vi "Configure.vi"(10 "CfgIn":T8={"Baud Rate"=enum."9600 bps", "Baud Rate Divider"=192, "Prescaler"=enum."1", "Data Bits"=enum."8", "Stop Bits"=enum."1", "Parity"=enum."None", "Flow Control"=enum."None", "Transceiver Mode"=enum."4 Wire"}, 11 "Serial FPGA in":refnum<class "Serial FPGA.lvclass">) -> (3 "Serial FPGA out":refnum<class "Serial FPGA.lvclass">)   [LabVIEW 2013, in "Serial FPGA.lvclass"]
uses:
  Serial FPGA.lvclass
  <vilib>/LabVIEW Targets/FPGA/cRIO/shared/nicrio_ModuleControls/nicrio_cRIO-9871_BaudRateEnum.ctl
  <vilib>/LabVIEW Targets/FPGA/cRIO/shared/nicrio_ModuleControls/nicrio_cRIO-9871_BaudRatePrescalerEnum.ctl
  <vilib>/LabVIEW Targets/FPGA/cRIO/shared/nicrio_ModuleControls/nicrio_cRIO-9871_DataBitsEnum.ctl
  <vilib>/LabVIEW Targets/FPGA/cRIO/shared/nicrio_ModuleControls/nicrio_cRIO-9871_StopBitsEnum.ctl
  <vilib>/LabVIEW Targets/FPGA/cRIO/shared/nicrio_ModuleControls/nicrio_cRIO-9871_ParityEnum.ctl
  <vilib>/LabVIEW Targets/FPGA/cRIO/shared/nicrio_ModuleControls/nicrio_cRIO-9871_FlowControlEnum.ctl
  <vilib>/LabVIEW Targets/FPGA/cRIO/shared/nicrio_ModuleControls/nicrio_cRIO-9871_XcvrModeEnum.ctl
  Serial FPGA.lvclass/Serial FPGA.ctl
  <vilib>/rvi/eio/common/nirviEmuTemplatePropertySet_noerrors.vi
  <vilib>/eio/EIOPropertyNode/EIOPropertyNode.xnode
  <vilib>/rvi/eio/common/nirviEmuTemplatePropertyGet_errors.vi
  <vilib>/rvi/eio/common/nirviEmuTemplatePropertyGet_noerrors.vi
  <vilib>/rvi/eio/common/nirviEmuTemplatePropertySet_errors.vi
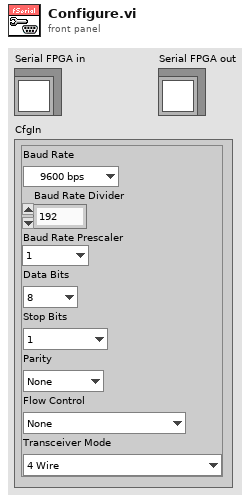
[diagram p1: front panel]
types:
  T1 = typedef "nicrio_cRIO-9871_BaudRateEnum.ctl" = enum16{"75 bps", "110 bps", "134 bps", "150 bps", "300 bps", "600 bps", "1200 bps", "1800 bps", "2400 bps", "4800 bps", "7200 bps", "9600 bps", "14.4 kbps", "19.2 kbps", "28.8 kbps", "38.4 kbps", "57.6 kbps", "115.2 kbps", "230.4 kbps", "460.8 kbps", "921.6 kbps"}
  T2 = typedef "nicrio_cRIO-9871_BaudRatePrescalerEnum.ctl" = enum8{"1", "4"}
  T3 = typedef "nicrio_cRIO-9871_DataBitsEnum.ctl" = enum8{"5", "6", "7", "8"}
  T4 = typedef "nicrio_cRIO-9871_StopBitsEnum.ctl" = enum8{"1", "1.5", "2"}
  T5 = typedef "nicrio_cRIO-9871_ParityEnum.ctl" = enum8{"None", "Odd", "Even", "Mark", "Space"}
  T6 = typedef "nicrio_cRIO-9871_FlowControlEnum.ctl" = enum8{"None", "Software (XON / XOFF)", "Hardware (RTS / CTS)"}
  T7 = typedef "nicrio_cRIO-9871_XcvrModeEnum.ctl" = enum8{"4 Wire", "2 Wire DTR Controlled with Echo", "2 Wire DTR Controlled", "2 Wire Auto"}
  T8 = cluster{"Baud Rate":T1, "Baud Rate Divider":u16, "Prescaler":T2, "Data Bits":T3, "Stop Bits":T4, "Parity":T5, "Flow Control":T6, "Transceiver Mode":T7}
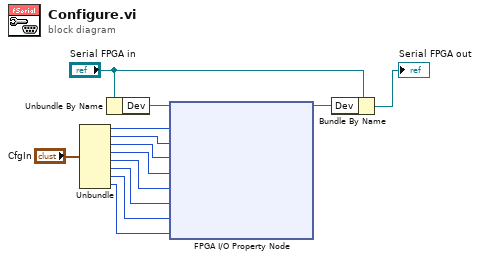
[diagram p0: block diagram]
diagram:
  n1 = Unbundle("CfgIn") -> ("Baud Rate"=w11:T1, "Baud Rate Divider"=w10:u16, "Prescaler"=w9:T2, "Data Bits"=w8:T3, "Stop Bits"=w7:T4, "Parity"=w6:T5, "Flow Control"=w5:T6, "Transceiver Mode"=w4:T7)
  n2 = Unbundle By Name("Serial FPGA in") -> ("Dev"=w13:refnum<k21>)
  n3 = xnode "FPGA I/O Property Node"("FPGA I/O In"=w13, "Baud Rate"=w11, "Baud Rate Divider"=w10, "Baud Rate Prescaler"=w9, "Data Bits"=w8, "Stop Bits"=w7, "Parity"=w6, "Flow Control"=w5, "Transceiver Mode"=w4) -> ("FPGA I/O Out"=w2:refnum<k21>)
  n4 = Bundle By Name(cluster="Serial FPGA in", "Dev"=w2) -> (→"Serial FPGA out":refnum<class "Serial FPGA.lvclass">)
